vi "CRYPART CLOSE FRAME.vi"(7 "sAction":string, 10 "tFrame":T2, 11 "nID":i32) -> ()   [LabVIEW 2013]
uses:
  <vilib>/Utility/miscctls.llb/LVRectTypeDef.ctl
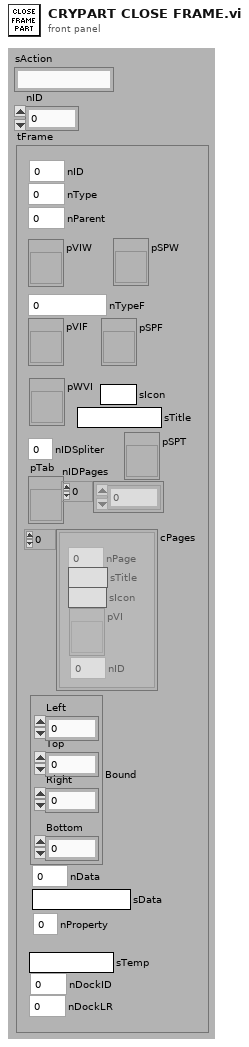
[diagram p1: front panel]
types:
  T1 = typedef "LVRectTypeDef.ctl" = cluster{"Left":i16, "Top":i16, "Right":i16, "Bottom":i16}
  T2 = cluster{"nType":i32, "nParent":i32, "pVIW":refnum<vi>, "pSPW":refnum<vi>, "nTypeF":i32, "pVIF":refnum<vi>, "pSPF":refnum<vi>, "nIDSpliter":i32, "nProperty":i32, "Bound":T1, "nID":i32, "nData":i32, "sData":string, "pWVI":refnum<vi>, "sTitle":string, "cPages":cluster{"nPage":i32, "sTitle":string, "sIcon":string, "pVI":refnum<vi>, "nID":i32}[], "pTab":refnum<vi>, "nIDPages":i32[], "pSPT":refnum<vi>, "sTemp":string, "nDockID":i32, "nDockLR":i32, "sIcon":string}
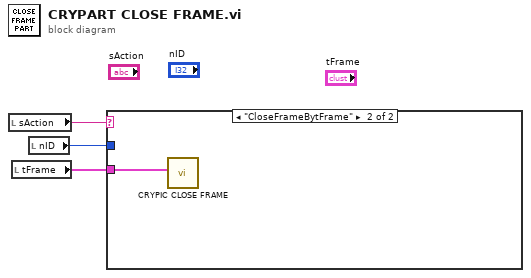
[diagram p0: block diagram]
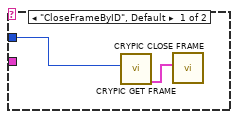
[diagram p2: hidden frame]
diagram:
  n1 = local read "sAction"() -> (w3:string)
  n2 = local read "tFrame"() -> (w2:T2)
  n3 = local read "nID"() -> (w1:i32)
  n4 = case shown="\"CloseFrameBytFrame\"" w3 {
    tunnel: w2 -> [_ w6]
    tunnel: w1 -> [w5 _]
    frame "CloseFrameByID", Default {
      n5 = call "CRYPIC GET FRAME.vi"("nID"=w5) -> ("tFrame_Out"=w4:T2)  [unwired: 8 in, 2 out]
      n6 = call "CRYPIC CLOSE FRAME.vi"("tFrame"=w4) -> ()  [unwired: 11 in]
    }
    frame "CloseFrameBytFrame" {
      n7 = call "CRYPIC CLOSE FRAME.vi"("tFrame"=w6) -> ()  [unwired: 11 in]
    }
  }
